vi "Read Server Address.vi"(8 "error in (no error)":errorcluster, 11 "Server Fixture in":refnum<class "Server Fixture.lvclass">) -> (0 "error out":errorcluster, 2 "Server Address":string, 3 "Server Fixture out":refnum<class "Server Fixture.lvclass">)   [LabVIEW 2013, in "libssh2_integration_tests.lvlib" / "Server Fixture.lvclass"]
uses:
  Server Fixture.lvclass
  Server Fixture.lvclass/Server Fixture.ctl
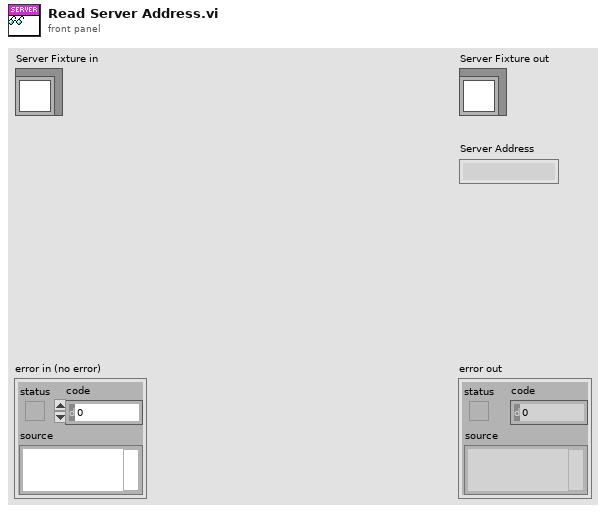
[diagram p1: front panel]
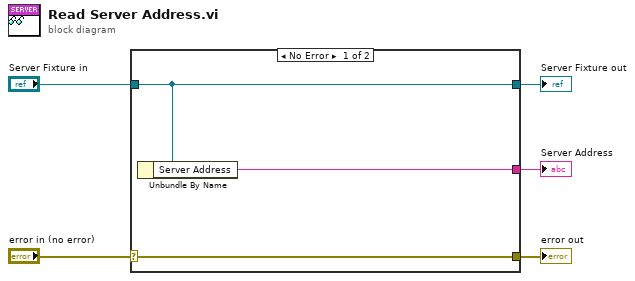
[diagram p0: block diagram]
diagram:
  n1 = case shown="No Error" "error in (no error)" {
    selector: "error in (no error)" -> [w8 w9]
    tunnel: [w8 w9] -> w4
    tunnel: [w7 w10] -> w2
    tunnel: "Server Fixture in" -> [w7 w10]
    tunnel: [w6 _] -> w1
    frame No Error {
      n2 = Unbundle By Name(w7) -> ("Server Address"=w6:string)
    }
    frame Error {
    }
  }
  "error out" <- w4
  "Server Fixture out" <- w2
  "Server Address" <- w1
